vi "AMC e.bloxx Get Device Status.vi"(8 "error in (no error)":errorcluster, 10 "Module Address":i32, 11 "VISA Resource Name":refnum<visa-resource-name>) -> (0 "error out":errorcluster, 1 "Module Status":i32, 2 "Channel Status":i32, 3 "VISA Resource Name out":refnum<visa-resource-name>)   [LabVIEW 2013]
doc: "<B>AMC - Analytik & Messtechnik GmbH Chemnitz</B>\n\nLabVIEW Drivers for e.bloxx series from Gantner Instruments\n\nThis VI reads the device status from the module specified by <B>Module Address</B>."
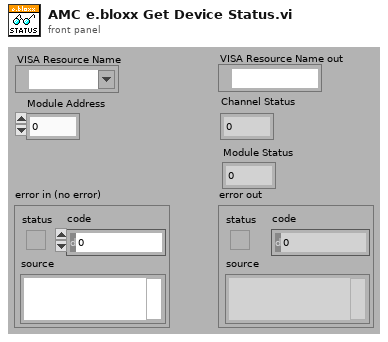
[diagram p1: front panel]
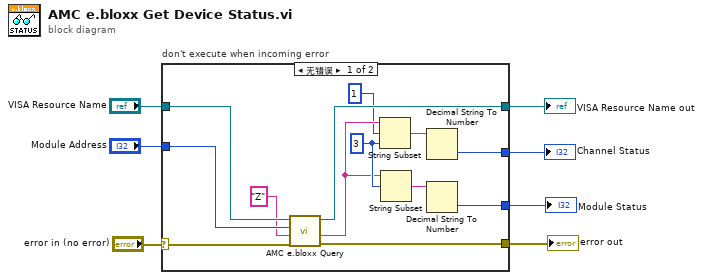
[diagram p0: block diagram]
diagram:
  n1 = case "don't execute when incoming error" shown="无错误" "error in (no error)" {
    selector: "error in (no error)" -> [w20 w22]
    tunnel: [w16 w22] -> w6
    tunnel: "VISA Resource Name" -> [w18 w21]
    tunnel: "Module Address" -> [w19 _]
    tunnel: [w15 w21] -> w3
    tunnel: [w13 _] -> w2
    tunnel: [w9 _] -> w1
    frame No Error {
      w12 = 3 ("length (rest)")
      n2 = call "AMC e.bloxx Query.vi"("error in (no error)"=w20, "Module Command"="Z", "Module Address"=w19, "VISA Resource Name"=w18) -> ("error out"=w16:errorcluster, "Module Response"=w11:string, "VISA Resource Name out"=w15:refnum<visa-resource-name>)  [unwired: 5 in]
      n3 = String Subset(string=w11, offset (0)=1, length (rest)=w12) -> (substring=w14:string)
      n4 = String Subset(string=w11, offset (0)=w12) -> (substring=w10:string)  [unwired: 1 in]
      n5 = Decimal String To Number(string=w14) -> (number=w13:i32)  [unwired: 2 in, 1 out]
      n6 = Decimal String To Number(string=w10) -> (number=w9:i32)  [unwired: 2 in, 1 out]
    }
    frame Error {
    }
  }
  "error out" <- w6
  "VISA Resource Name out" <- w3
  "Channel Status" <- w2
  "Module Status" <- w1
